vi "READ HV SUPPLIES.vi"(0 "ORSAY":refnum<visa-resource-name>, 2 "HV SUPPLY":u16(ring) items=["BEAM ENERGY", "EXTRACTOR", "SUPPRESSOR", "CONDENSOR", "OBJECTIVE"], 11 "ORSAY ERROR":errorcluster, 12 "APPEND":string) -> (4 "ORSAY 2":refnum<visa-resource-name>, 6 "VOLTAGE":dbl[unit], 8 "CURRENT":dbl[unit], 15 "ORSAY ERROR":errorcluster)   [LabVIEW 2018]
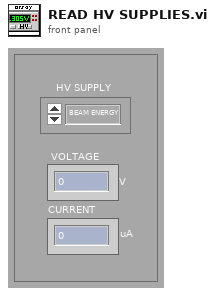
[diagram p1: front panel]
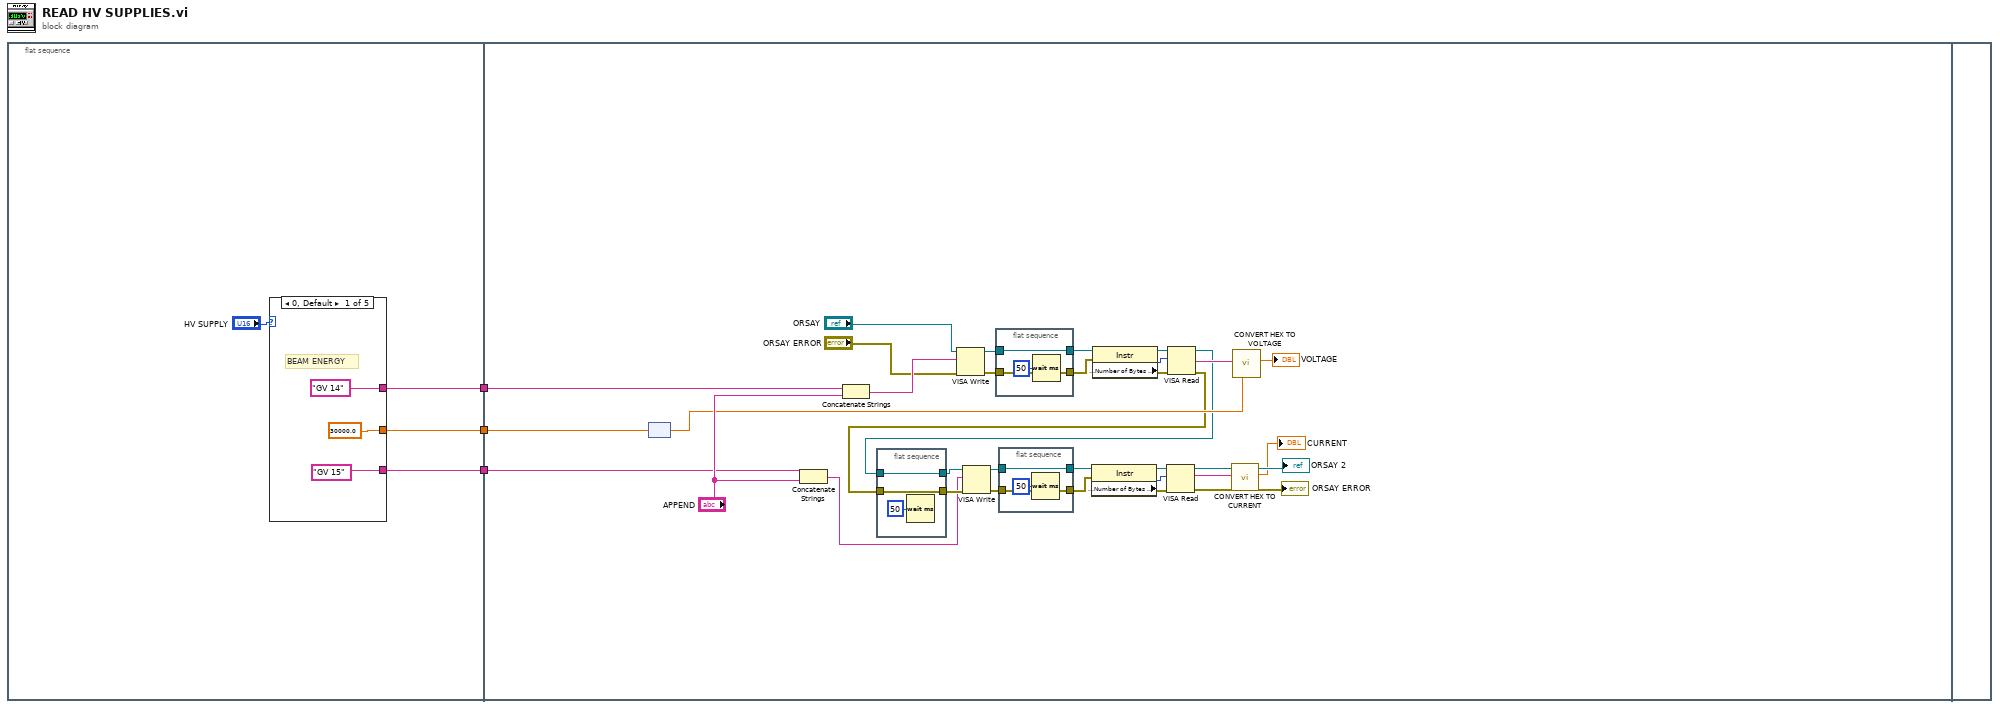
[diagram p0: block diagram]
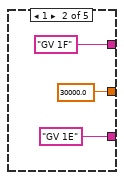
[diagram p2: hidden frame]
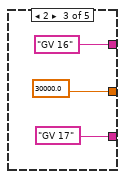
[diagram p3: hidden frame]
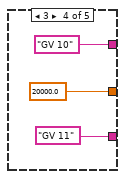
[diagram p4: hidden frame]
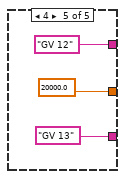
[diagram p5: hidden frame]
diagram:
  n1 = flat-sequence {
    tunnel: [w7] -> w3
    tunnel: [w6] -> w2
    tunnel: [w5] -> w1
    tunnel: w3 -> [w52]
    tunnel: w2 -> [w51]
    tunnel: w1 -> [w49]
    frame #0 {
      n2 = case shown="0, Default" "HV SUPPLY" {
        tunnel: ["GV 14" "GV 1F" "GV 16" "GV 10" "GV 12"] -> w7
        tunnel: [sgl 30000.0 ("Max supply") sgl 30000.0 ("Max supply") 30000.0 ("Max supply") 20000.0 ("Max supply") 20000.0 ("Max supply")] -> w6
        tunnel: ["GV 15" "GV 1E" "GV 17" "GV 11" "GV 13"] -> w5
        frame 0, Default {
          # "BEAM ENERGY"
        }
        frame 1 {
        }
        frame 2 {
        }
        frame 3 {
        }
        frame 4 {
        }
      }
    }
    frame #1 {
      n3 = node(w51) -> (w50:dbl[unit])
      n4 = Concatenate Strings(w49, "APPEND") -> (w23:string)
      n5 = Concatenate Strings(w52, "APPEND") -> (w48:string)
      n6 = flat-sequence {
        tunnel: [w58] -> w26
        tunnel: w27 -> [w58]
        tunnel: [w57] -> w25
        tunnel: w24 -> [w57]
        frame #0 {
          n7 = Wait (ms)(milliseconds to wait=u32 50) -> ()  [unwired: 1 out]
        }
      }
      n8 = VISA Write(VISA resource name="ORSAY", write buffer=w48, error in (no error)="ORSAY ERROR") -> (VISA resource name out=w42:refnum<visa-resource-name>, error out=w41:errorcluster)  [unwired: 1 out]
      n9 = VISA Write(VISA resource name=w26, write buffer=w23, error in (no error)=w25) -> (VISA resource name out=w35:refnum<visa-resource-name>, error out=w34:errorcluster)  [unwired: 1 out]
      n10 = flat-sequence {
        tunnel: w42 -> [w63]
        tunnel: w41 -> [w62]
        tunnel: [w63] -> w46
        tunnel: [w62] -> w47
        frame #0 {
          n11 = Wait (ms)(milliseconds to wait=u32 50) -> ()  [unwired: 1 out]
        }
      }
      n12 = flat-sequence {
        tunnel: w35 -> [w60]
        tunnel: w34 -> [w59]
        tunnel: [w60] -> w39
        tunnel: [w59] -> w40
        frame #0 {
          n13 = Wait (ms)(milliseconds to wait=u32 50) -> ()  [unwired: 1 out]
        }
      }
      n14 = property class="Instr"(reference=w39, error in=w40) -> (reference out=w36:refnum<visa-resource-name>, error out=w37:errorcluster, "Serial Settings:Number of Bytes at Serial Port"=w38:u32)
      n15 = property class="Instr"(reference=w46, error in=w47) -> (reference out=w43:refnum<visa-resource-name>, error out=w44:errorcluster, "Serial Settings:Number of Bytes at Serial Port"=w45:u32)
      n16 = VISA Read(VISA resource name=w36, byte count=w38, error in (no error)=w37) -> (VISA resource name out=→"ORSAY 2":refnum<visa-resource-name>, read buffer=w32:string, error out=→"ORSAY ERROR":errorcluster)  [unwired: 1 out]
      n17 = VISA Read(VISA resource name=w43, byte count=w45, error in (no error)=w44) -> (VISA resource name out=w27:refnum<visa-resource-name>, read buffer=w33:string, error out=w24:errorcluster)  [unwired: 1 out]
      n18 = call "CONVERT HEX TO CURRENT.vi"("HEX STRING"=w32) -> ("CURRENT"=→"CURRENT":dbl[unit])  [unwired: 10 in]
      n19 = call "CONVERT HEX TO VOLTAGE.vi"("SUPPLY RANGE"=w50, "HEX STRING"=w33) -> ("x/y"=→"VOLTAGE":dbl[unit])  [unwired: 9 in]
    }
    frame #2 {
    }
  }
